vi "ezAFM Practice 1.1.vi"() -> ()   [LabVIEW 2015]
uses:
  D:/LabVIEW for ezAFM/LV-PGC 2019-05a/Special Equipment/ezAFM/NMI Integration Code/ezCommander.dll
  LabVIEW for ezAFM/LV-PGC 2019-05a/Special Equipment/ezAFM/NMI Integration Code/ezCommander.dll
panel:
  in  "MOVE":bool
  out "Move2Device Vector":dbl[](array[numeric])
  in  "THETA":bool
  in  "Move2Device":string(combo)
  in  "Angle":dbl
  in  "RESET":bool
  out "ezAFM Connected":bool
  in  "QUIT":bool
  out "XY Position":dbl[](array[numeric])
  out "Status":string
  in  "Step Size":dbl
  in  "Motor Speed":dbl
  in  "LEFT":bool
  in  "RIGHT":bool
  in  "DOWN":bool
  in  "UP":bool
  # "Navigation Buttons"
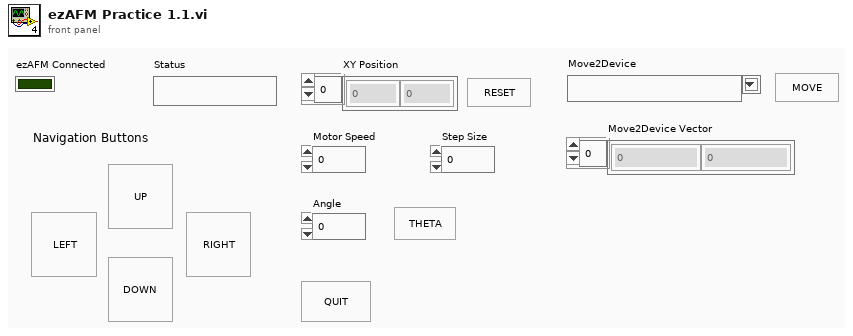
[diagram p1: front panel]
types:
  T1 = typedef "eventvkey.ctl" = enum16{"ASCII", "Enter", "Return", "Shift", "Ctrl", "Alt", "Cmd", "Opt", "Caps", "NumLock", "Clear", "Break", "Up", "Down", "Left", "Right", "Insert", "Delete", "Home", "End", "PageUp", "PageDown", "Escape", "Help", "Pause", "ScrollLock", "F1", "F2", "F3", "F4", "F5", "F6", "F7", "F8", "F9", "F10", "F11", "F12", "F13", "F14", "F15", "F16", "F17", "F18", "F19", "F20", "F21", "F22", "F23", "F24", "Play", "VolumeUp", "VolumeDown", "Mute", "Two Byte Char"}
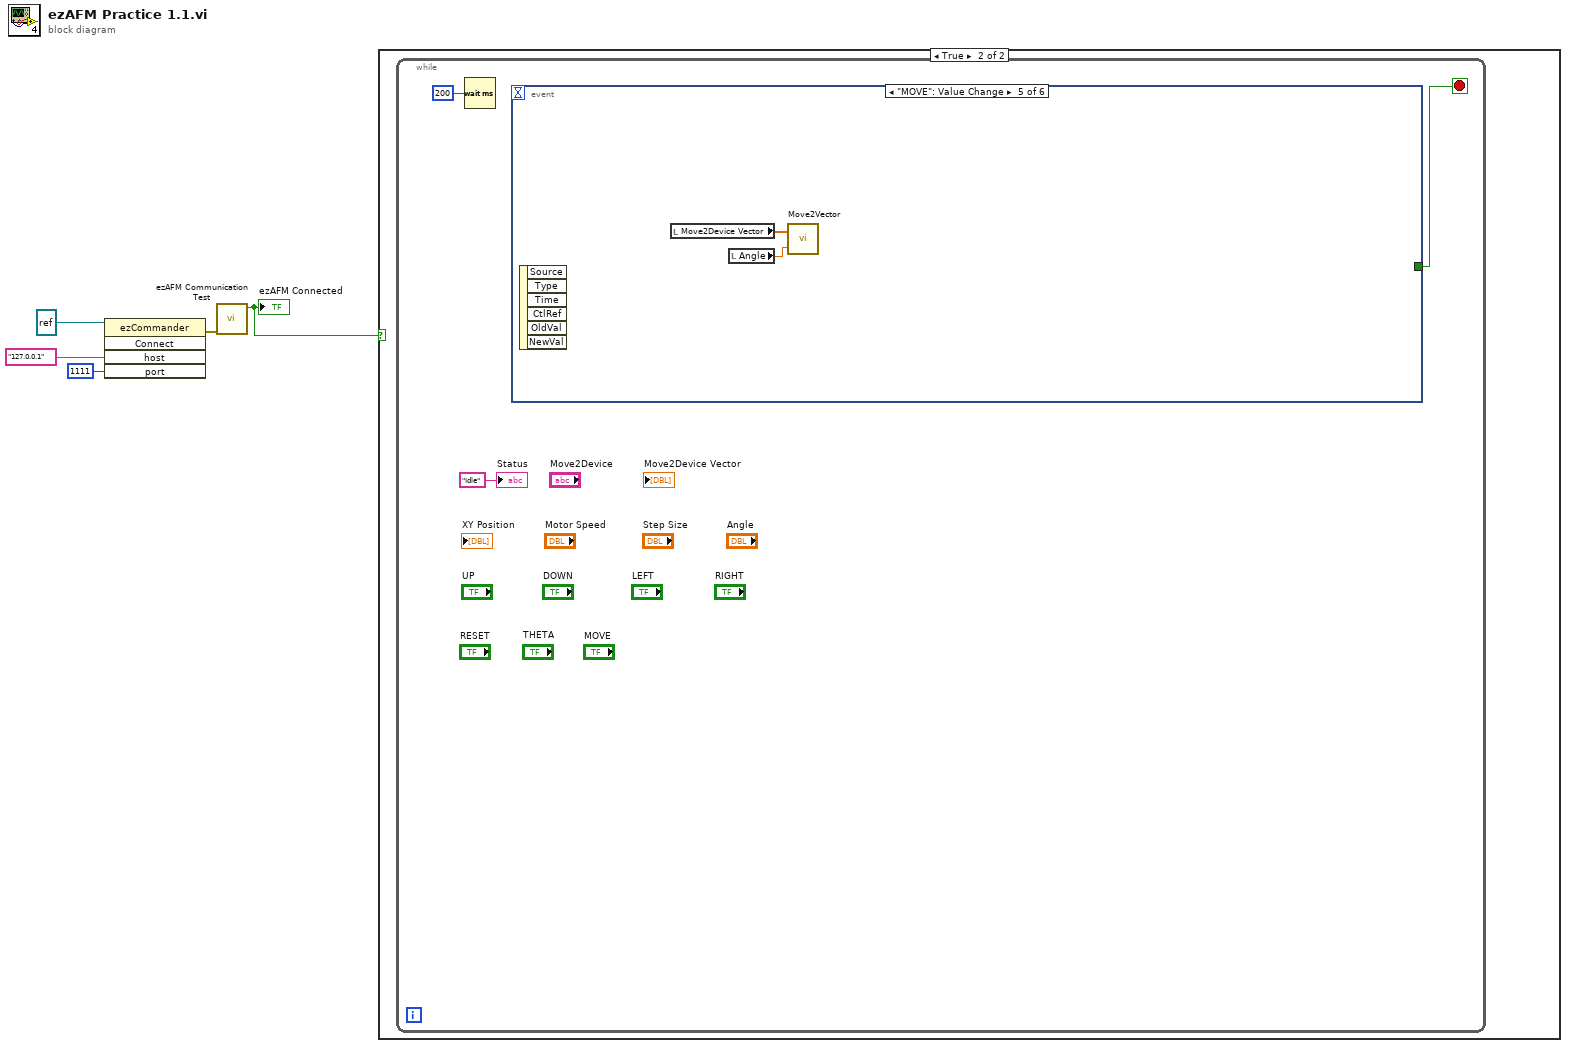
[diagram p0: block diagram]
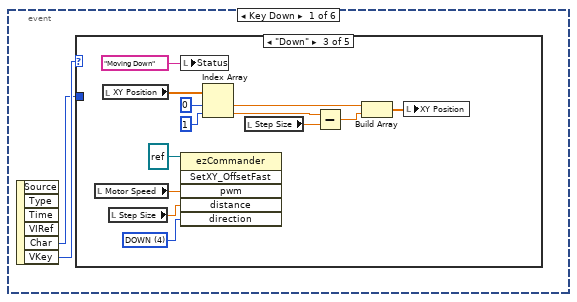
[diagram p3: hidden frame]
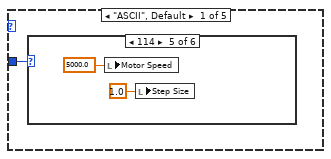
[diagram p4: hidden frame]
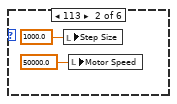
[diagram p6: hidden frame]
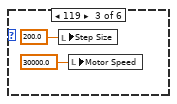
[diagram p7: hidden frame]
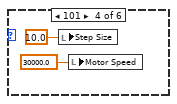
[diagram p8: hidden frame]
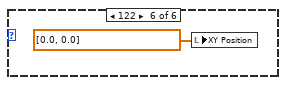
[diagram p9: hidden frame]
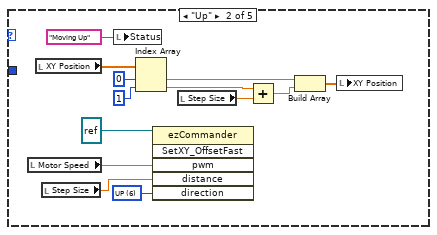
[diagram p10: hidden frame]
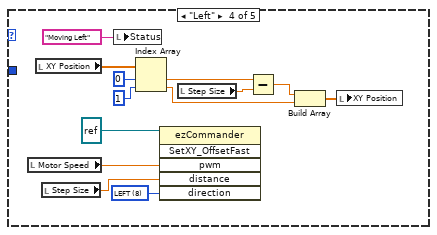
[diagram p11: hidden frame]
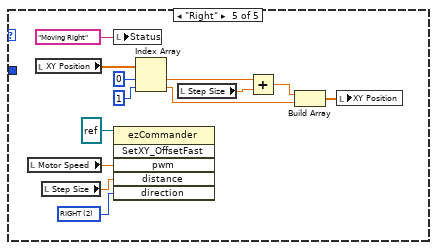
[diagram p12: hidden frame]
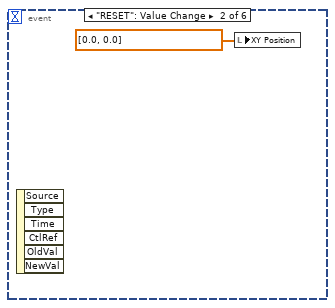
[diagram p13: hidden frame]
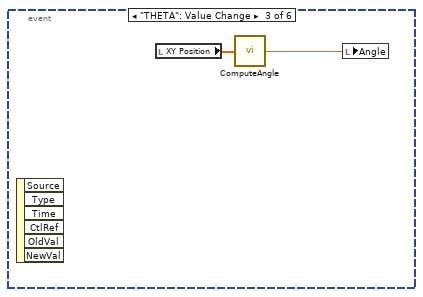
[diagram p14: hidden frame]
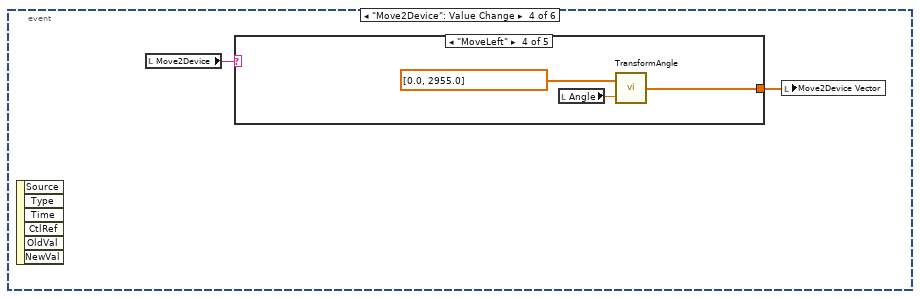
[diagram p15: hidden frame]
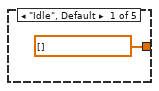
[diagram p16: hidden frame]
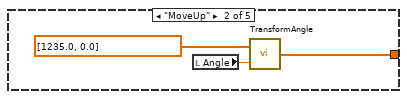
[diagram p17: hidden frame]
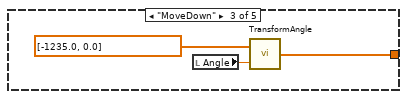
[diagram p18: hidden frame]
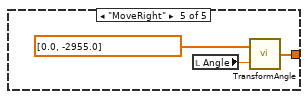
[diagram p19: hidden frame]
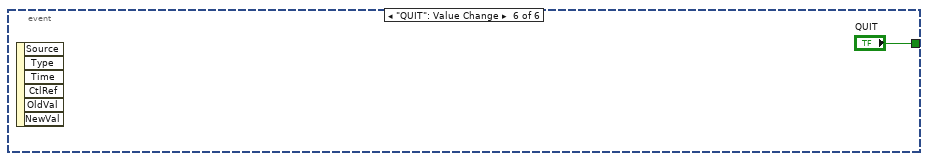
[diagram p20: hidden frame]
diagram:
  n1 = invoke class="ezCommander" method="Connect"(reference=refnum<k24> refnum ("ezAFM Ref"), "host"="127.0.0.1", "port"=1111) -> (error out=w4:errorcluster)  [unwired: 2 in, 4 out]
  n2 = call "ezAFM Communication Test.vi"("error in"=w4) -> ("ezAFM COM status"=w1:bool)  [unwired: 3 in, 3 out]
  "ezAFM Connected" <- w1
  n3 = case shown="True" w1 {
    frame False {
    }
    frame True {
      n4 = while {
        stop <- w8 stop-if-true
        n5 = Wait (ms)(milliseconds to wait=u32 200) -> ()  [unwired: 1 out]
        n6 = event shown="[4] \"MOVE\": Value Change" {
          selector: _ -> [_ _ _ _ _ _]
          dyn-events: _ -> [_ _ _ _ _ _]
          timeout: _ -> [_ _ _ _ _ _]
          tunnel: [_ _ _ _ _ "QUIT"] -> w8
          event Key Down {
            n7 = event-data() -> ("Char"=w9:i16, "VKey"=w10:T1)  [unwired: 1 in, 4 out]
            n8 = case shown="\"Down\"" w10 {
              tunnel: w9 -> [w11 _ _ _ _]
              frame "ASCII", Default {
                n9 = case shown="114" w11 {
                  frame 0, Default {
                  }
                  frame 113 {
                    n10 = local write "Step Size"(1000.0 ("Step Size")) -> ()
                    n11 = local write "Motor Speed"(50000.0 ("Motor Speed")) -> ()
                  }
                  frame 119 {
                    n12 = local write "Step Size"(200.0 ("Step Size")) -> ()
                    n13 = local write "Motor Speed"(30000.0 ("Motor Speed")) -> ()
                  }
                  frame 101 {
                    n14 = local write "Step Size"(10.0 ("Step Size")) -> ()
                    n15 = local write "Motor Speed"(30000.0 ("Motor Speed")) -> ()
                  }
                  frame 114 {
                    n16 = local write "Motor Speed"(5000.0 ("Motor Speed")) -> ()
                    n17 = local write "Step Size"(1.0 ("Step Size")) -> ()
                  }
                  frame 122 {
                    n18 = local write "XY Position"(dbl[] [0.0, 0.0] ("XY Position")) -> ()
                  }
                }
              }
              frame "Up" {
                w31 = u16 6 items=["UP"=6, "DOWN"=4, "LEFT"=8, "RIGHT"=2]
                n19 = local read "Motor Speed"() -> (w30:dbl)
                n20 = local read "XY Position"() -> (w28:dbl[])
                n21 = local read "Step Size"() -> (w29:dbl)
                n22 = local write "Status"("Moving Up" ("Status")) -> ()
                n23 = Index Array(array=w28, index #1=0 ("index"), index #2=1 ("index")) -> (element #1=w23:dbl, element #2=w24:dbl)
                n24 = invoke class="ezCommander" method="SetXY_OffsetFast"(reference=refnum<k24> refnum ("ezAFM Ref"), "pwm"=w30, "distance"=w29, "direction"=w31) -> ()  [unwired: 2 in, 6 out]
                n25 = local read "Step Size"() -> (w25:dbl)
                n26 = Add(x=w24, y=w25) -> (x+y=w22:dbl)
                n27 = Build Array(w23, w22) -> (w21:dbl[])
                n28 = local write "XY Position"(w21) -> ()
              }
              frame "Down" {
                w43 = u16 4 items=["UP"=6, "DOWN"=4, "LEFT"=8, "RIGHT"=2]
                n29 = local read "Motor Speed"() -> (w45:dbl)
                n30 = local read "XY Position"() -> (w36:dbl[])
                n31 = local read "Step Size"() -> (w44:dbl)
                n32 = local write "Status"("Moving Down" ("Status")) -> ()
                n33 = invoke class="ezCommander" method="SetXY_OffsetFast"(reference=refnum<k24> refnum ("ezAFM Ref"), "pwm"=w45, "distance"=w44, "direction"=w43) -> ()  [unwired: 2 in, 6 out]
                n34 = Index Array(array=w36, index #1=0 ("index"), index #2=1 ("index")) -> (element #1=w38:dbl, element #2=w39:dbl)
                n35 = local read "Step Size"() -> (w35:dbl)
                n36 = Subtract(x=w39, y=w35) -> (x-y=w37:dbl)
                n37 = Build Array(w38, w37) -> (w34:dbl[])
                n38 = local write "XY Position"(w34) -> ()
              }
              frame "Left" {
                w58 = u16 8 items=["UP"=6, "DOWN"=4, "LEFT"=8, "RIGHT"=2]
                n39 = local read "Motor Speed"() -> (w56:dbl)
                n40 = local read "XY Position"() -> (w51:dbl[])
                n41 = local read "Step Size"() -> (w57:dbl)
                n42 = local write "Status"("Moving Left" ("Status")) -> ()
                n43 = Index Array(array=w51, index #1=0 ("index"), index #2=1 ("index")) -> (element #1=w49:dbl, element #2=w47:dbl)
                n44 = invoke class="ezCommander" method="SetXY_OffsetFast"(reference=refnum<k24> refnum ("ezAFM Ref"), "pwm"=w56, "distance"=w57, "direction"=w58) -> ()  [unwired: 2 in, 6 out]
                n45 = local read "Step Size"() -> (w52:dbl)
                n46 = Subtract(x=w49, y=w52) -> (x-y=w48:dbl)
                n47 = Build Array(w48, w47) -> (w50:dbl[])
                n48 = local write "XY Position"(w50) -> ()
              }
              frame "Right" {
                w71 = u16 2 items=["UP"=6, "DOWN"=4, "LEFT"=8, "RIGHT"=2]
                n49 = local read "Motor Speed"() -> (w70:dbl)
                n50 = local read "XY Position"() -> (w64:dbl[])
                n51 = local read "Step Size"() -> (w69:dbl)
                n52 = local write "Status"("Moving Right" ("Status")) -> ()
                n53 = invoke class="ezCommander" method="SetXY_OffsetFast"(reference=refnum<k24> refnum ("ezAFM Ref"), "pwm"=w70, "distance"=w69, "direction"=w71) -> ()  [unwired: 2 in, 6 out]
                n54 = Index Array(array=w64, index #1=0 ("index"), index #2=1 ("index")) -> (element #1=w62:dbl, element #2=w60:dbl)
                n55 = local read "Step Size"() -> (w63:dbl)
                n56 = Add(x=w62, y=w63) -> (x+y=w61:dbl)
                n57 = Build Array(w61, w60) -> (w65:dbl[])
                n58 = local write "XY Position"(w65) -> ()
              }
            }
          }
          event "RESET": Value Change {
            n59 = event-data() -> ()  [unwired: 1 in, 6 out]
            n60 = local write "XY Position"(dbl[] [0.0, 0.0] ("XY Position")) -> ()
          }
          event "THETA": Value Change {
            n61 = event-data() -> ()  [unwired: 1 in, 6 out]
            n62 = local read "XY Position"() -> (w75:dbl[])
            n63 = call "ComputeAngle.vi"("XY Vector"=w75) -> ("Angle"=w74:dbl)
            n64 = local write "Angle"(w74) -> ()
          }
          event "Move2Device": Value Change {
            n65 = event-data() -> ()  [unwired: 1 in, 6 out]
            n66 = local read "Move2Device"() -> (w77:string)
            n67 = case shown="\"MoveLeft\"" w77 {
              tunnel: [dbl[] [] w79 w82 w86 w89] -> w76
              frame "Idle", Default {
              }
              frame "MoveUp" {
                n68 = local read "Angle"() -> (w81:dbl)
                n69 = call "TransformAngle.vi"("Angle"=w81, "XY Vector"=dbl[] [1235.0, 0.0]) -> ("Result Vector"=w79:dbl[])
              }
              frame "MoveDown" {
                n70 = local read "Angle"() -> (w83:dbl)
                n71 = call "TransformAngle.vi"("Angle"=w83, "XY Vector"=dbl[] [-1235.0, 0.0]) -> ("Result Vector"=w82:dbl[])
              }
              frame "MoveLeft" {
                n72 = local read "Angle"() -> (w85:dbl)
                n73 = call "TransformAngle.vi"("Angle"=w85, "XY Vector"=dbl[] [0.0, 2955.0]) -> ("Result Vector"=w86:dbl[])
              }
              frame "MoveRight" {
                n74 = local read "Angle"() -> (w88:dbl)
                n75 = call "TransformAngle.vi"("Angle"=w88, "XY Vector"=dbl[] [0.0, -2955.0]) -> ("Result Vector"=w89:dbl[])
              }
            }
            n76 = local write "Move2Device Vector"(w76) -> ()
          }
          event "MOVE": Value Change {
            n77 = event-data() -> ()  [unwired: 1 in, 6 out]
            n78 = local read "Move2Device Vector"() -> (w91:dbl[])
            n79 = local read "Angle"() -> (w92:dbl)
            n80 = call "Move2Vector.vi"("Angle"=w92, "XY Vector"=w91) -> ()  [unwired: 1 in]
          }
          event "QUIT": Value Change {
            n81 = event-data() -> ()  [unwired: 1 in, 6 out]
          }
        }
        "Status" <- "Idle" ("Status")
      }
    }
  }
